vi "search-double.vi"(10 "Search":dbl=nan format="%#_13g", 11 "Data (dbl) []":dbl[](array[numeric])) -> (2 "Index":i32)   [LabVIEW 2015, in "binary_search.lvlib"]
uses:
  binary_search.lvlib
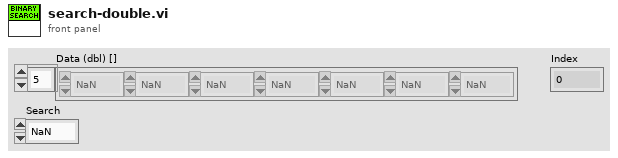
[diagram p1: front panel]
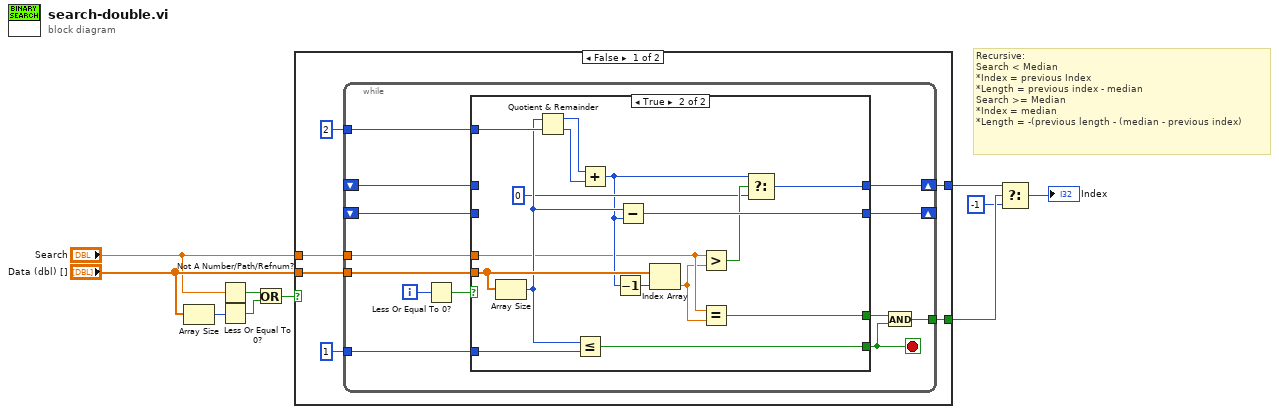
[diagram p0: block diagram]
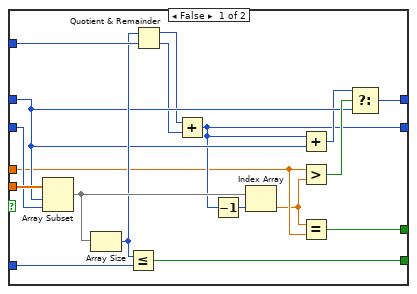
[diagram p2: hidden frame]
diagram:
  # "Recursive:\nSearch < Median\n*Index = previous Index\n*Length = previous index - median\nSearch >= Median\n*Index = median\n*Length = -(previous length - (median - previous index)"
  n1 = Array Size(array="Data (dbl) []") -> (size(s)=w6:i32)
  n2 = Not A Number/Path/Refnum?(number/path/refnum="Search") -> (NaN/Path/Refnum?=w10:bool)
  n3 = Less Or Equal To 0?(x=w6) -> (x <= 0?=w9:bool)
  n4 = Or(x=w10, y=w9) -> (x .or. y?=w1:bool)
  n5 = case shown="False" w1 {
    tunnel: "Data (dbl) []" -> [w16 _]
    tunnel: "Search" -> [w15 _]
    tunnel: [w12 _] -> w5
    tunnel: [w11 _] -> w4
    frame False {
      n6 = while {
        tunnel: w16 -> [w27]
        tunnel: w15 -> [w29]
        shift-right: [w26] -> w11
        shift-left: _ -> [w28]
        shift-right: [w25] -> _
        shift-left: _ -> [w24]
        tunnel: 1 ("y") -> [w21]
        tunnel: 2 ("y") -> [w20]
        tunnel: [w17] -> w12
        i -> [w23]
        stop <- w18 stop-if-true
        n7 = Less Or Equal To 0?(x=w23) -> (x <= 0?=w22:bool)
        n8 = case shown="True" w22 {
          tunnel: w29 -> [w34 w51]
          tunnel: w28 -> [w38 _]
          tunnel: w27 -> [w47 w63]
          tunnel: [w43 w60] -> w26
          tunnel: [w35 w62] -> w25
          tunnel: w24 -> [w46 _]
          tunnel: [w32 w49] -> w18
          tunnel: w21 -> [w44 w59]
          tunnel: w20 -> [w41 w58]
          tunnel: [w30 w48] -> w19
          frame False {
            n9 = Array Subset(array=w47, index=w38, length=w46) -> (w45:dbl[])
            n10 = Array Size(array=w45) -> (size(s)=w40:i32)
            n11 = Less Or Equal?(x=w40, y=w44) -> (x <= y?=w32:bool)
            n12 = Quotient & Remainder(x=w40, y=w41) -> (x-y*floor(x/y)=w36:i32, floor(x/y)=w31:i32)
            n13 = Add(x=w36, y=w31) -> (x+y=w35:i32)
            n14 = Decrement(x=w35) -> (x-1=w39:i32)
            n15 = Index Array(array=w45, index=w39) -> (element=w33:dbl)
            n16 = Add(x=w35, y=w38) -> (x+y=w37:i32)
            n17 = Greater?(x=w34, y=w33) -> (0:w42:bool)
            n18 = Equal?(x=w33, y=w34) -> (x = y?=w30:bool)
            n19 = Select(t=w37, s=w42, f=w38) -> (s? t:f=w43:i32)
          }
          frame True {
            n20 = Array Size(array=w63) -> (size(s)=w57:i32)
            n21 = Quotient & Remainder(x=w57, y=w58) -> (x-y*floor(x/y)=w52:i32, floor(x/y)=w54:i32)
            n22 = Less Or Equal?(x=w57, y=w59) -> (x <= y?=w49:bool)
            n23 = Add(x=w52, y=w54) -> (x+y=w53:i32)
            n24 = Decrement(x=w53) -> (x-1=w55:i32)
            n25 = Subtract(x=w57, y=w53) -> (x-y=w62:i32)
            n26 = Index Array(array=w63, index=w55) -> (element=w50:dbl)
            n27 = Greater?(x=w51, y=w50) -> (0:w61:bool)
            n28 = Equal?(x=w51, y=w50) -> (x = y?=w48:bool)
            n29 = Select(t=w53, s=w61, f=0) -> (s? t:f=w60:i32)
          }
        }
        n30 = And(x=w19, y=w18) -> (x .and. y?=w17:bool)
      }
    }
    frame True {
    }
  }
  n31 = Select(t=w4, s=w5, f=-1) -> (s? t:f=→"Index":i32)
